vi "WPI_SimpleGyro_Close.vi"(8 "error in":errorcluster, 11 "SimpleGyroDevRef":T1) -> (0 "error out":errorcluster)   [LabVIEW 2015, in "SimpleGyro.lvlib"]
doc: "Closes the SimpleGyroDevRef and properly shuts down SPI communication between the RoboRIO and the SimpleGyro."
uses:
  SimpleGyro.lvlib
  WPI_SimpleGyroDevRef.ctl
  <vilib>/Rock Robotics/SystemInterfaces/spilib/spi_bus.ctl
  <vilib>/Rock Robotics/WPI/SPI/WPI_SPIDevRef.ctl
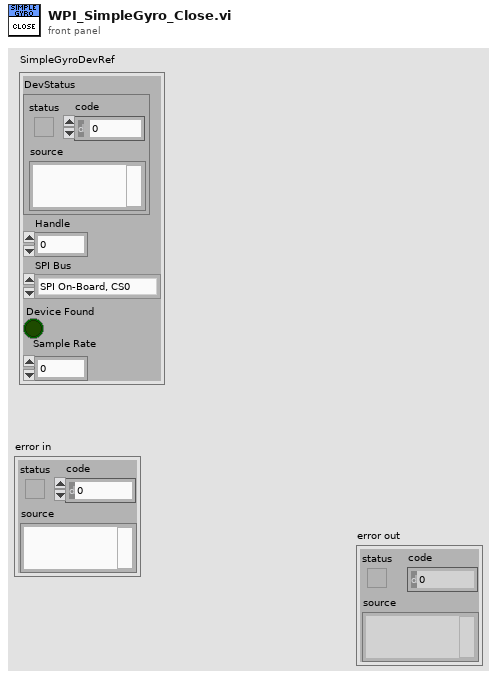
[diagram p1: front panel]
types:
  T1 = typedef "SimpleGyro.lvlib/WPI_SimpleGyroDevRef.ctl" = cluster{"DevStatus":errorcluster, "Handle":i32, "SPI Bus":T2, "Device Found":bool, "Sample Rate":dbl}
  T2 = typedef "spi_bus.ctl" = enum16{"SPI On-Board, CS0", "SPI On-Board, CS1", "SPI On-Board, CS2", "SPI On-Board, CS3", "SPI MXP", "Invalid"}
  T3 = typedef "WPI_SPIDevRef.ctl" = cluster{"DevStatus":errorcluster, "Handle":i32, "SPI Bus":T2}
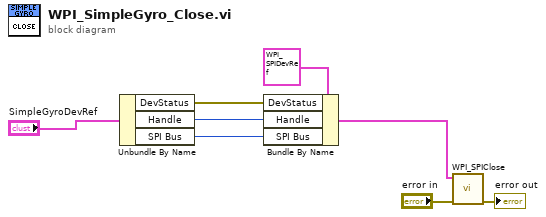
[diagram p0: block diagram]
diagram:
  n1 = Unbundle By Name("SimpleGyroDevRef") -> ("DevStatus"=w4:errorcluster, "Handle"=w3:i32, "SPI Bus"=w2:T2)
  n2 = Bundle By Name(cluster=T3 {"DevStatus"={"status"=FALSE, "code"=0, "source"=""}, "Handle"=0, "SPI Bus"=enum."SPI On-Board, CS0"} ("SPIDevRef"), "DevStatus"=w4, "Handle"=w3, "SPI Bus"=w2) -> (w1:T3)
  n3 = call <vilib>:"WPI_SPIClose.vi"("error in (no error)"="error in", "SPIDevRef"=w1) -> ("error out"=→"error out":errorcluster)  [unwired: 9 in]
